vi "getState.vi"(8 "error in (no error)":errorcluster, 11 "FaultState in":refnum<class "FaultState.lvclass">) -> (0 "error out":errorcluster, 2 "DeviceStatus":T1, 3 "FaultState out":refnum<class "FaultState.lvclass">)   [LabVIEW 2016, in "FaultState.lvclass"]
uses:
  FaultState.lvclass
  Typedefs/DeviceStatus.ctl
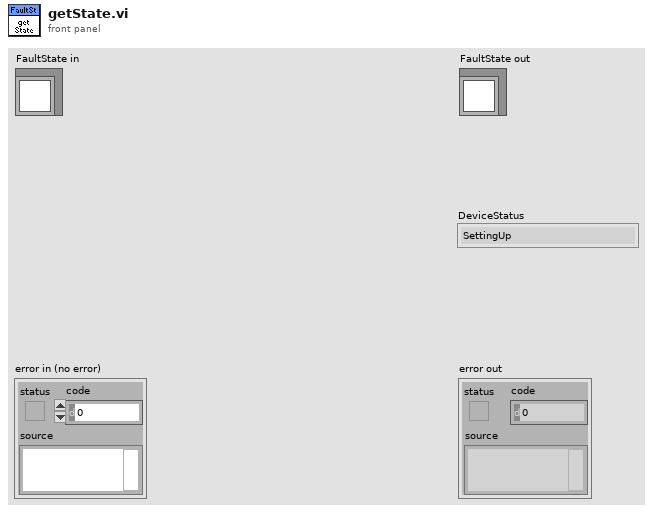
[diagram p1: front panel]
types:
  T1 = typedef "DeviceStatus.ctl" = enum16{"SettingUp", "Ready", "Offline", "Fault"}
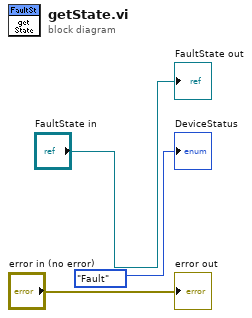
[diagram p0: block diagram]
diagram:
  "error out" <- "error in (no error)"
  "FaultState out" <- "FaultState in"
  "DeviceStatus" <- DeviceStatus."Fault" ("DeviceStatus")
